vi "Parse Launch Parameters.vi"(3 "DB Data":string[][](array[string])) -> (1 "Processes to Launch":T1[](array[typedef]))   [LabVIEW 2020, in "Config Data.lvlib" / "Config Data_DB_ADO.lvclass"]
uses:
  Config Data_DB_ADO.lvclass
  typedefs/Process Launch Data.ctl
  typedefs/Process Type.ctl
  Config Data.lvclass
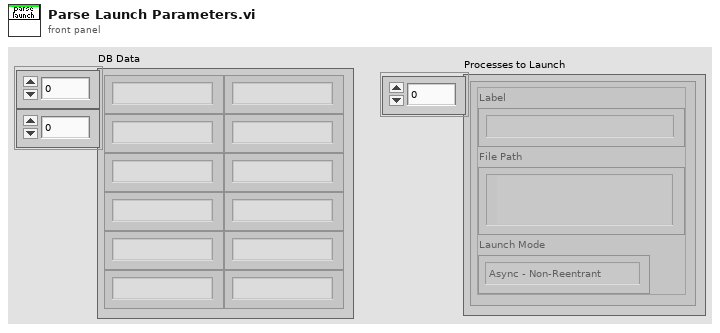
[diagram p1: front panel]
types:
  T1 = typedef "Config Data.lvlib/Config Data.lvclass/Process Launch Data.ctl" = cluster{"Label":string, "File Path":path, "Launch Mode":T2}
  T2 = typedef "Config Data.lvlib/Config Data.lvclass/Process Type.ctl" = enum16{"Async - Non-Reentrant", "Async - Reentrant", "Run Method - Non-Reentrant", "Run Method - Reentrant"}
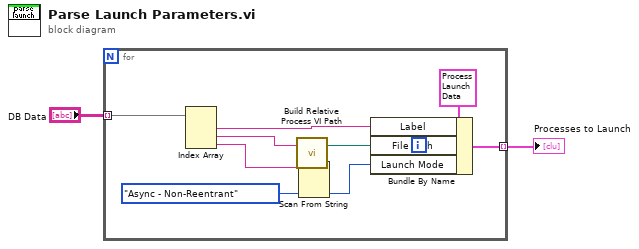
[diagram p0: block diagram]
diagram:
  n1 = for {
    tunnel: [w10] -> w2 mode=indexing
    tunnel: "DB Data" -> [w9] mode=indexing
    n2 = Index Array(array=w9) -> (element #1=w8:string, element #2=w4:string, element #3=w7:string)  [unwired: 3 in]
    n3 = call "Build Relative Process VI Path.vi"("Rel Path"=w4) -> ("Full Path Out"=w3:path)  [unwired: 2 in]
    n4 = Scan From String(input string=w7, default 1=Process_Type."Async - Non-Reentrant" ("Launch Mode")) -> (output 1=w5:T2)  [unwired: 3 in, 3 out]
    n5 = Bundle By Name(cluster=T1 {"Label"="", "File Path"=path "", "Launch Mode"=enum."Async - Non-Reentrant"} ("Cluster"), "Label"=w8, "File Path"=w3, "Launch Mode"=w5) -> (w10:T1)
  }
  "Processes to Launch" <- w2
